vi "EXA_getNextSample_Summary.vi"(8 "error in (no error)":errorcluster, 11 "Summary_Ctl":T1={"EXAmple[16]"=[FALSE, FALSE, FALSE, FALSE, FALSE, FALSE, FALSE, FALSE, FALSE, FALSE, FALSE, FALSE, FALSE, FALSE, FALSE, FALSE]}) -> (0 "error out":errorcluster, 2 "function return":i32, 3 "Summary_Ctl out":T1)   [LabVIEW 2016, in "SALLV_EXA.lvlib"]
doc: "int EXA_shm_getNextSample_SummaryLV(EXA_SummaryLV *Summary_Ctl );"
uses:
  SALLV_EXA.lvlib
  DataTypes/Summary.ctl
  SALLV_EXA.so
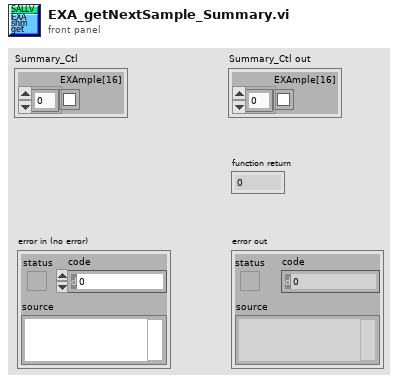
[diagram p1: front panel]
types:
  T1 = typedef "SALLV_EXA.lvlib/Summary.ctl" = cluster{"EXAmple[16]":bool[]}
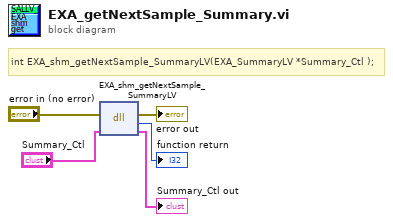
[diagram p0: block diagram]
diagram:
  # "int EXA_shm_getNextSample_SummaryLV(EXA_SummaryLV *Summary_Ctl );"
  n1 = dll-call lib="home/plotz/SALLV_EXA/SALLV_EXA.*" fn="EXA_shm_getNextSample_SummaryLV"(error in="error in (no error)", "Summary_Ctl"="Summary_Ctl") -> (error out=→"error out":errorcluster, →"function return":i32, "Summary_Ctl"=→"Summary_Ctl out":T1)  [unwired: 2 in, 1 out]
